vi "Event Msg To Nested.vi"(8 "Alias":string, 10 "Msg":refnum<class "Msg.lvclass">, 11 "jettl Queue Actor in":refnum<class "jettl Queue Actor.lvclass">) -> (0 "error out":errorcluster)   [LabVIEW 2021, in "jettl.lvlib" / "jettl Queue Actor.lvlib" / "jettl Queue Actor.lvclass"]
uses:
  jettl Queue Actor.lvclass
  Actor/Msg/Msg.lvclass
  jettl Queue Actor.lvclass/jettl Queue Actor.ctl
  jettl.lvlib
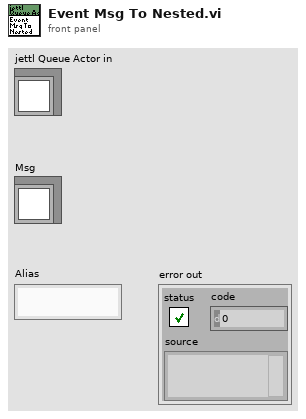
[diagram p1: front panel]
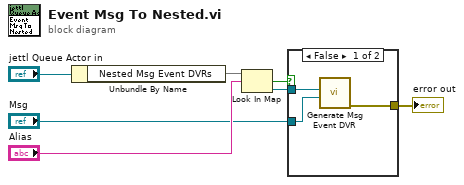
[diagram p0: block diagram]
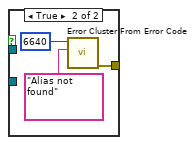
[diagram p2: hidden frame]
diagram:
  n1 = Unbundle By Name("jettl Queue Actor in") -> ("Nested Msg Event DVRs"=w6:map{string, refnum<data-value>})
  n2 = Look In Map(map=w6, key="Alias") -> (key not found?=w4:bool, value=w3:refnum<data-value>)  [unwired: 1 in]
  n3 = case shown="False" w4 {
    tunnel: [w8 w13] -> w1
    tunnel: "Msg" -> [w9 _]
    tunnel: w3 -> [w10 _]
    frame False {
      n4 = call "Generate Msg Event DVR.vi"("Msg"=w9, "Msg Event DVR"=w10) -> ("error out"=w8:errorcluster)  [unwired: 9 in]
    }
    frame True {
      n5 = call <vilib>:"Error Cluster From Error Code.vi"("error message (\"\")"="Alias not found" ("error message (\"\")"), "error code (0)"=6640) -> ("error out"=w13:errorcluster)  [unwired: 7 in]
    }
  }
  "error out" <- w1
